vi "DisplayBoard.vi"(8 "error in (no error)":errorcluster, 10 "GameRecorder":refnum<class "GameRecorder.lvclass">, 11 "BoardDisplay in":refnum<class "BoardDisplay.lvclass">) -> (0 "error out":errorcluster, 2 "BoardVisulalization":picture[][](array[picture]), 3 "BoardDisplay out":refnum<class "BoardDisplay.lvclass">)   [LabVIEW 2015, in "TronviewPresentation.lvlib" / "BoardDisplay.lvclass"]
uses:
  BoardDisplay.lvclass
  TronviewGame/GameRecorder/GameRecorder.lvclass
  TrajectoryBoardField.ctl
  TrajectoryFieldType.ctl
  TronVIEWBotAPI/MovementDirection.ctl
  TronviewGame/GameRecorder/GameRecorder.lvclass/GameRecorder.ctl
  TronviewGame/Board/Board.lvclass/Board.ctl
  TronviewGame/GameRecorder/GetPlayer1Moves.vi
  TronviewGame/GameRecorder/GetInitialBoard.vi
  TronviewGame/GameRecorder/GetPlayer2Moves.vi
  TronviewGame/Board/GetSize.vi
  TronviewGame/Board/GetPlayer1Position.vi
  TronviewGame/Board/GetPlayer2Position.vi
  TronviewGame/Board/FindFieldPosition.vi
  TronviewGame/Board/Board.lvclass
  TronVIEWBotAPI/TronVIEWBotAPI.lvlib
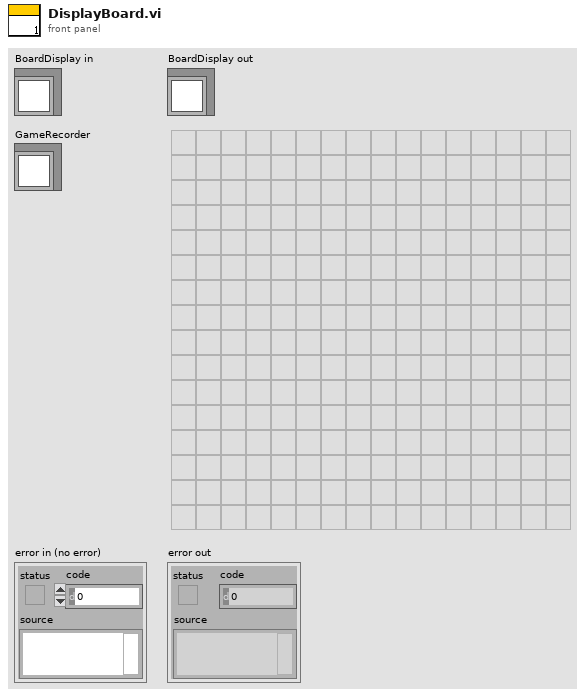
[diagram p1: front panel]
types:
  T1 = typedef "TronviewPresentation.lvlib/BoardDisplay.lvclass/TrajectoryBoardField.ctl" = cluster{"FieldType":T2, "Player":string, "ComingFrom":T3, "GoingTo":T3}
  T2 = typedef "TronviewPresentation.lvlib/BoardDisplay.lvclass/TrajectoryFieldType.ctl" = enum16{"Empty", "Initial", "PlayerWall", "PlayerPosition"}
  T3 = typedef "TronVIEWBotAPI.lvlib/MovementDirection.ctl" = enum16{"N", "S", "W", "E"}
  T4 = typedef "TronviewGame.lvlib/Board.lvclass/BoardSize.ctl" = cluster{"Columns":u16, "Rows":u16}
  T5 = typedef "TronviewGame.lvlib/Board.lvclass/Position.ctl" = cluster{"Column":i32, "Row":i32}
  T6 = typedef "TronviewPresentation.lvlib/BoardDisplay.lvclass/PlayerTrajectory.ctl" = cluster{"Field":T5, "ComingFrom":T3, "GoingTo":T3}
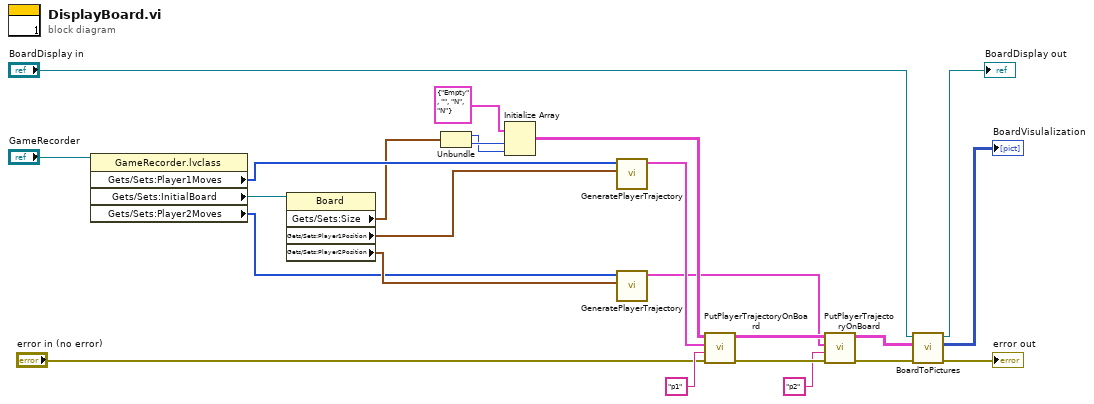
[diagram p0: block diagram]
diagram:
  n1 = property class="GameRecorder.lvclass"(reference="GameRecorder") -> ("Gets/Sets:Player1Moves"=w21:T3[], "Gets/Sets:InitialBoard"=w23:refnum<class "Board.lvclass">, "Gets/Sets:Player2Moves"=w16:T3[])  [unwired: 1 in, 2 out]
  n2 = property class="Board"(reference=w23) -> ("Gets/Sets:Size"=w18:T4, "Gets/Sets:Player1Position"=w22:T5, "Gets/Sets:Player2Position"=w17:T5)  [unwired: 1 in, 2 out]
  n3 = Unbundle(w18) -> ("Columns"=w19:u16, "Rows"=w20:u16)
  n4 = Initialize Array(T1 {"FieldType"=enum."Empty", "Player"="", "ComingFrom"=enum."N", "GoingTo"=enum."N"} ("TrajectoryBoardField"), w20, w19) -> (w13:T1[][])
  n5 = call "GeneratePlayerTrajectory.vi"("InitialPlayerPosition"=w22, "PlayerMoves"=w21) -> ("PlayerTrajectory"=w14:T6[])  [unwired: 9 in]
  n6 = call "GeneratePlayerTrajectory.vi"("InitialPlayerPosition"=w17, "PlayerMoves"=w16) -> ("PlayerTrajectory"=w9:T6[])  [unwired: 9 in]
  n7 = call "PutPlayerTrajectoryOnBoard.vi"("error in (no error)"="error in (no error)", "PlayerID"="p1", "PlayerTrajectory"=w14, "Board in"=w13) -> ("error out"=w11:errorcluster, "Board out"=w10:T1[][])  [unwired: 6 in]
  n8 = call "PutPlayerTrajectoryOnBoard.vi"("error in (no error)"=w11, "PlayerID"="p2", "PlayerTrajectory"=w9, "Board in"=w10) -> ("error out"=w4:errorcluster, "Board out"=w2:T1[][])  [unwired: 6 in]
  n9 = call "BoardToPictures.vi"("error in (no error)"=w4, "Board"=w2, "BoardDisplay in"="BoardDisplay in") -> ("error out"=→"error out":errorcluster, "BoardVisulalization"=→"BoardVisulalization":picture[][], "BoardDisplay out"=→"BoardDisplay out":refnum<class "BoardDisplay.lvclass">)  [unwired: 6 in]
